vi "control_loop.vi"() -> ()   [LabVIEW 2022 SP3]
uses:
  <vilib>/Simulation/Scripting/Companion Diagram/SimConfigNode/SimDog.xnode
  <vilib>/Simulation/Implementation/Shared/SIMSCR Execution Mode.ctl
  <vilib>/Simulation/Scripting/Companion Diagram/SimConfigNode/_simSolvers.ctl
  <vilib>/Simulation/Scripting/Companion Diagram/SimConfigNode/SimParams.ctl
  <vilib>/Simulation/ContinuousLinear/Implementation/NILVSim Integrator new.llb/SIM Integrator (scalar).vi
  <vilib>/Simulation/Implementation/XNodeFramework/SimXNode/SimX.xnode
  <vilib>/Simulation/SignalArithmetic/Implementation/NILVSim Gain.llb/SIM Gain (scalar).vi
  <vilib>/Simulation/ContinuousLinear/Implementation/NILVSim Derivative.llb/SIM derivative (scalar).vi
  <vilib>/Simulation/DataSources/Implementation/NILVSim Step.llb/SIM Step (scalar).vi
  <vilib>/Simulation/Utility/Implementation/SIM Time.vi
  <vilib>/Simulation/SignalDisplay/Implementation/NILVSim Time Waveform.llb/SIM Time Waveform (scalar).vi
  <vilib>/Simulation/DataSources/Implementation/NILVSim Sine Wave.llb/SIM Sine Wave (scalar).vi
  <vilib>/Simulation/DataSources/Implementation/NILVSim Chirp Signal.llb/SIM Chirp Signal (scalar).vi
  <vilib>/Simulation/Implementation/Shared/SIM Bundle Sim Info.vi
  <vilib>/Simulation/Implementation/Shared/SIM Unbundle Sim Info.vi
  <vilib>/Simulation/Implementation/Shared/NILVSim_FinalizeModel.vi
  <vilib>/Simulation/Implementation/Shared/NILVSim_GetModelError.vi
  <vilib>/Simulation/Implementation/Shared/NILVSim_Initialize.vi
  <vilib>/Simulation/Utility/Implementation/NILVSim Get Time and IsAcceptedStep.vi
  <vilib>/Simulation/Implementation/Shared/NILVSim_Manager.vi
  <vilib>/Simulation/Implementation/Shared/NI_SIM_Implementation.lvlib
  <vilib>/Simulation/Implementation/Shared/NILVSIM_BeginStep.vi
  <vilib>/Simulation/Param Hierarchy/Typedefs/SIMPH Param Control Actions.ctl
  <vilib>/Simulation/Implementation/Shared/NILVSim_ParamChanged.vi
  <vilib>/Utility/error.llb/Clear Errors.vi
  <vilib>/Simulation/Implementation/Shared/SIMSH Read Queue.vi
  <vilib>/Simulation/ContinuousLinear/Implementation/NILVSim Integrator new.llb/SIM Integrator distributor (scalar).vi
  <vilib>/Simulation/ContinuousLinear/Implementation/NILVSim Integrator new.llb/SIM Integrator collector (scalar).vi
  <vilib>/Simulation/Implementation/Shared/SIM limit type.ctl
  <vilib>/Simulation/Implementation/Shared/SIM Is Init or Final Stage.vi
panel:
  out "body pos":waveform(dbl)(graph)
  out "entry":waveform(dbl)(graph)
  out "Ride Comfort Index":dbl(knob) scale=0.1..100.0
  in  "PID Switch":bool
  out "Simulation Running":bool
  out "Simulation Time (s)":dbl
  out "Tire Acc (m/s²)":dbl
  out "Body Acc (m/s²)":dbl
  out "Tire Position":dbl(graph)
  out "Body Position":dbl(graph)
  out "Body Velocity":dbl(graph)
  out "Input":dbl(graph)
  in  "STOP SIMULATION":bool
  in  "Road Input Type":T1(ring)
  in  "Ct (N,s/m)":dbl
  in  "Kt (N/m)":dbl
  in  "Cs (N,s/m)":dbl
  in  "Ks (N/m)":dbl
  in  "mu (kg)":dbl
  in  "ms (Kg)":dbl format="%#_350g"
  in  "Kd":dbl(knob) scale=0.0..100000.0
  in  "Ki":dbl(knob) scale=0.0..50.0
  in  "Kp":dbl(knob) scale=0.0..50.0
  # "Active Suspension Control System"
  # "OUTPUT GRAPHS"
  # "INDICATORS"
  # "PID CONTROLS"
  # "System Parameter Controls"
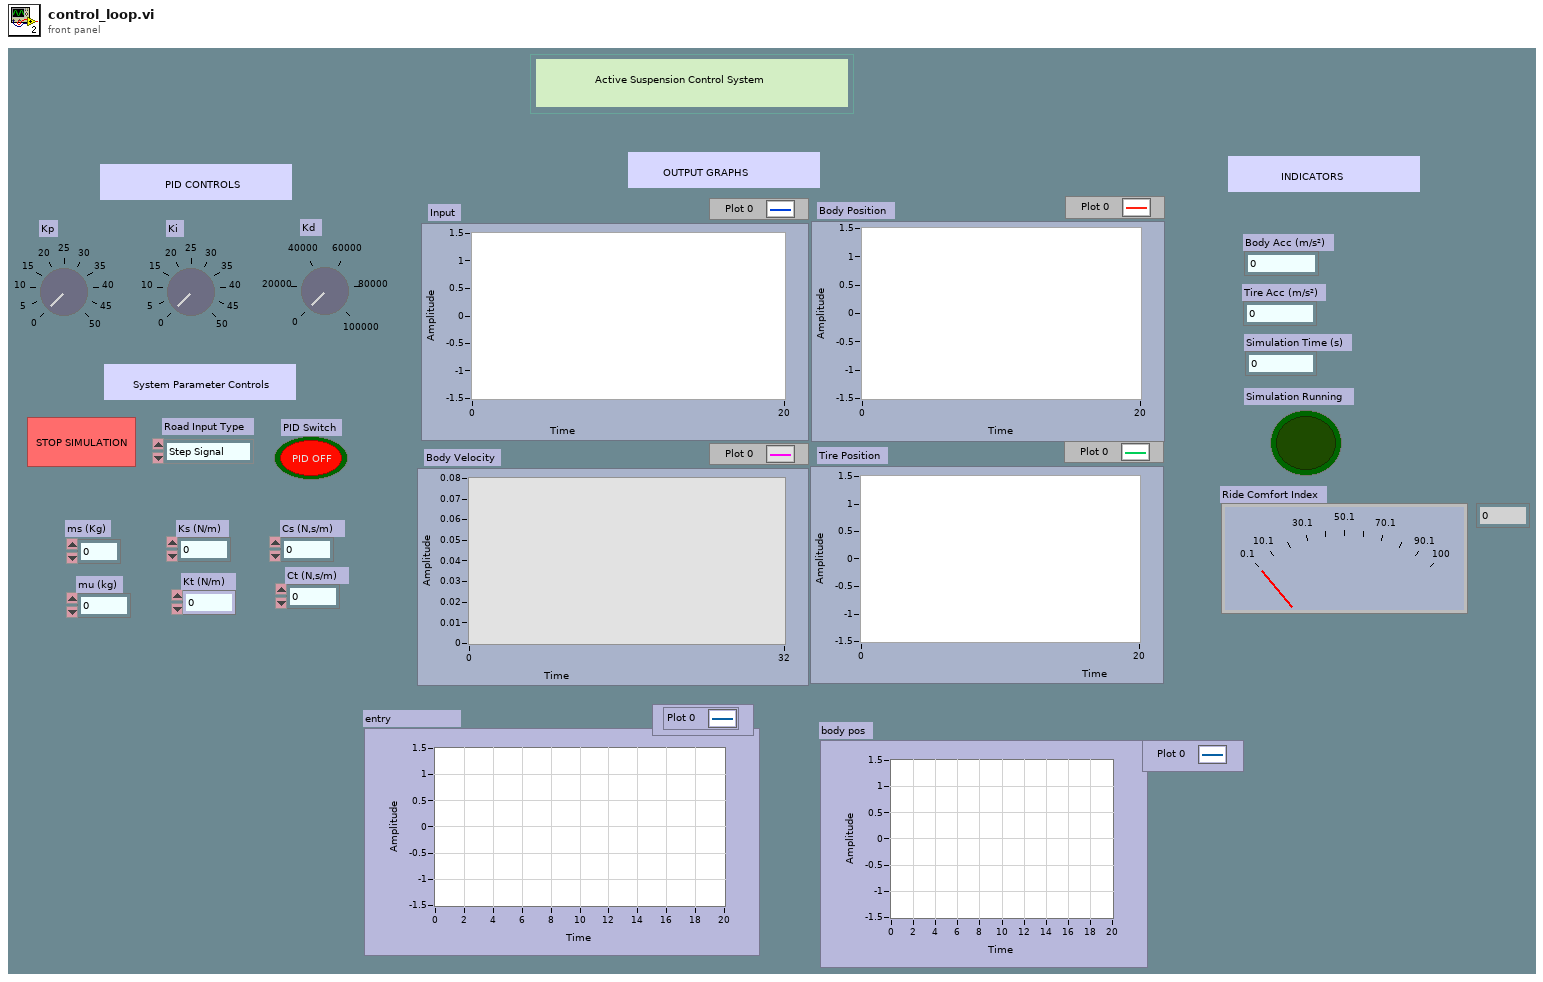
[diagram p1: front panel]
types:
  T1 = enum16{"Step Signal", "Sine Signal", "Chirp Signal"}
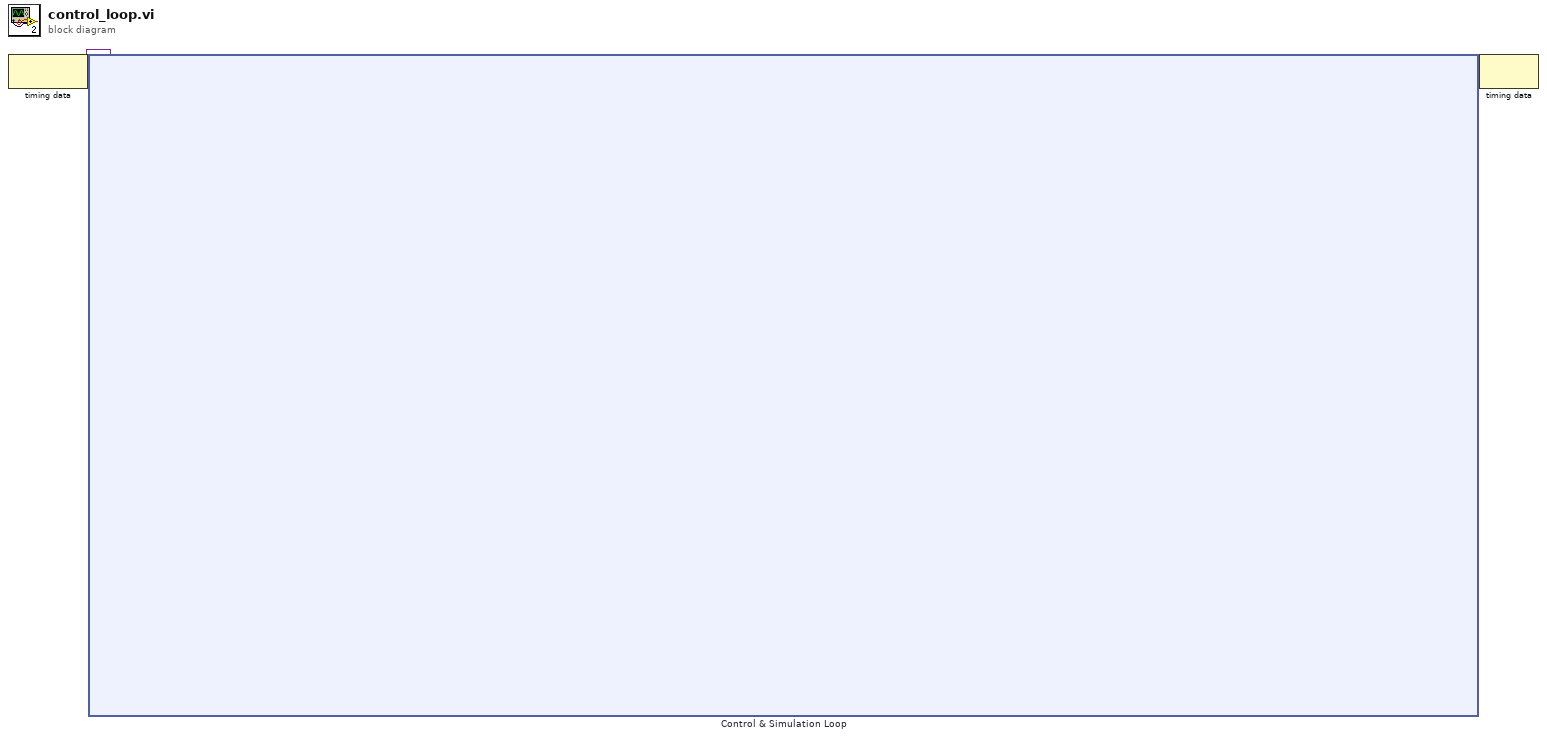
[diagram p0: block diagram]
diagram:
  n1 = node-c288() -> (w2:variant)  [unwired: 1 in]
  n2 = node-c254 "Control & Simulation Loop"(w2) -> (w1:variant)
  n3 = node-c288(w1) -> ()  [unwired: 1 out]
